vi "Read Ignore Timestamp.vi"(9 "WaveformGraph in":refnum<class "WaveformGraph.lvclass">) -> (3 "WaveformGraph out":refnum<class "WaveformGraph.lvclass">, 4 "Ignore Timestamp":bool)   [LabVIEW 2014, in "WaveformGraph.lvclass"]
uses:
  WaveformGraph.lvclass
  WaveformGraph.lvclass/WaveformGraph.ctl
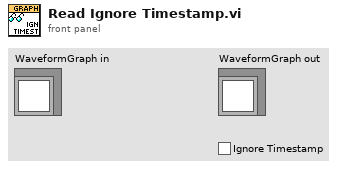
[diagram p1: front panel]
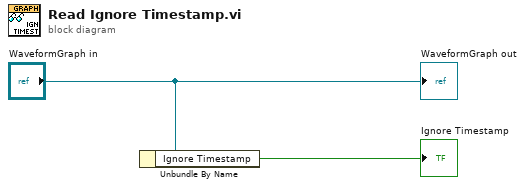
[diagram p0: block diagram]
diagram:
  n1 = Unbundle By Name("WaveformGraph in") -> ("Ignore Timestamp"=→"Ignore Timestamp":bool)
  "WaveformGraph out" <- "WaveformGraph in"
